vi "Write Param.vi"(8 "error in (no error)":errorcluster, 10 "Param":refnum<class "Param.lvclass">, 11 "MB_TCP in":refnum<class "WebSocket Client CR.lvclass">) -> (0 "error out":errorcluster, 3 "MB_TCP out":refnum<class "WebSocket Client CR.lvclass">)   [LabVIEW 2021, in "WebSockets.lvlib" / "WebSocket Client CR.lvclass"]
uses:
  WebSocket Client CR.lvclass
  Master CR/Param/Param.lvclass
  WebSocket Client CR.lvclass/WebSocket Client CR.ctl
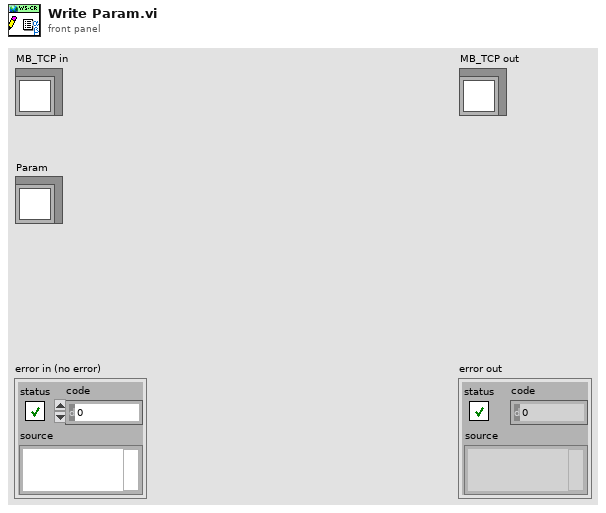
[diagram p1: front panel]
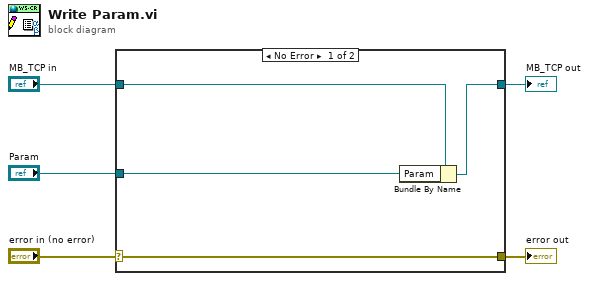
[diagram p0: block diagram]
diagram:
  n1 = case shown="No Error" "error in (no error)" {
    selector: "error in (no error)" -> [w9 w10]
    tunnel: [w9 w10] -> w4
    tunnel: [w7 w11] -> w2
    tunnel: "MB_TCP in" -> [w8 w11]
    tunnel: "Param" -> [w6 _]
    frame No Error {
      n2 = Bundle By Name(cluster=w8, "Param"=w6) -> (w7:refnum<class "WebSocket Client CR.lvclass">)
    }
    frame Error {
    }
  }
  "error out" <- w4
  "MB_TCP out" <- w2
